vi "two_button.vi"(7 "callee":refnum<vi>, 8 "error in (no error)":errorcluster, 11 "configuration":T1) -> (0 "error out":errorcluster, 3 "dialog_selection":T2)   [LabVIEW 2015, in "lv-dialog-interfaces.lvlib"]
uses:
  lv-dialog-interfaces.lvlib
  <userlib>/antonio-alexander/lv-dialog/api/v1/public/_controls/selection.ctl
  private/_controls/dialog_type.ctl
  private/_controls/hmi_references.ctl
  private/_controls/configuration.ctl
  <vilib>/event_ctls.llb/eventvkey.ctl
  <userlib>/antonio-alexander/lv-dialog/api/v1/v1.lvlib
panel:
  out "dialog":string
  in  "button_1":bool
  in  "button_2":bool
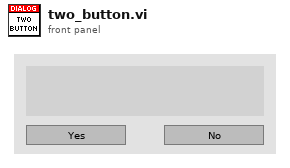
[diagram p1: front panel]
types:
  T1 = cluster{"dialog_text":string, "boolean_text_1":string, "boolean_text_2":string}
  T2 = typedef "lv-dialog.lvlib/v1.lvlib/selection.ctl" = enum16{"null", "panel_closed", "button_1", "button_2", "button_3", "cancelled"}
  T3 = typedef "lv-dialog-interfaces.lvlib/dialog_type.ctl" = enum16{"null", "one_button", "two_button", "three_button", "confirmation", "busy_wait", "error", "busy_wait_embed", "combo_box", "data_entry_string", "data_entry_numeric"}
  T4 = typedef "lv-dialog-interfaces.lvlib/configuration.ctl" = cluster{"dialog_text":string, "boolean_text_1":string, "boolean_text_2":string, "boolean_text_3":string, "inner_color":u32, "outer_color":u32, "wait_s":dbl, "error_status":bool, "error_source":string, "error_details":string, "string []":string[], "custom_entry":bool}
  T5 = typedef "lv-dialog-interfaces.lvlib/hmi_references.ctl" = cluster{"vi_reference":refnum<vi>, "caller":refnum<vi>, "dialog":refnum<vi>, "button_1":refnum<vi>, "button_2":refnum<vi>, "button_3":refnum<vi>, "busy":refnum<vi>, "error_glyph":refnum<vi>, "error_source":refnum<vi>, "error_text":refnum<vi>, "combo_box":refnum<vi>}
  T6 = typedef "eventvkey.ctl" = enum16{"ASCII", "Enter", "Return", "Shift", "Ctrl", "Alt", "Cmd", "Opt", "Caps", "NumLock", "Clear", "Break", "Up", "Down", "Left", "Right", "Insert", "Delete", "Home", "End", "PageUp", "PageDown", "Escape", "Help", "Pause", "ScrollLock", "F1", "F2", "F3", "F4", "F5", "F6", "F7", "F8", "F9", "F10", "F11", "F12", "F13", "F14", "F15", "F16", "F17", "F18", "F19", "F20", "F21", "F22", "F23", "F24", "Play", "VolumeUp", "VolumeDown", "Mute", "Two Byte Char"}
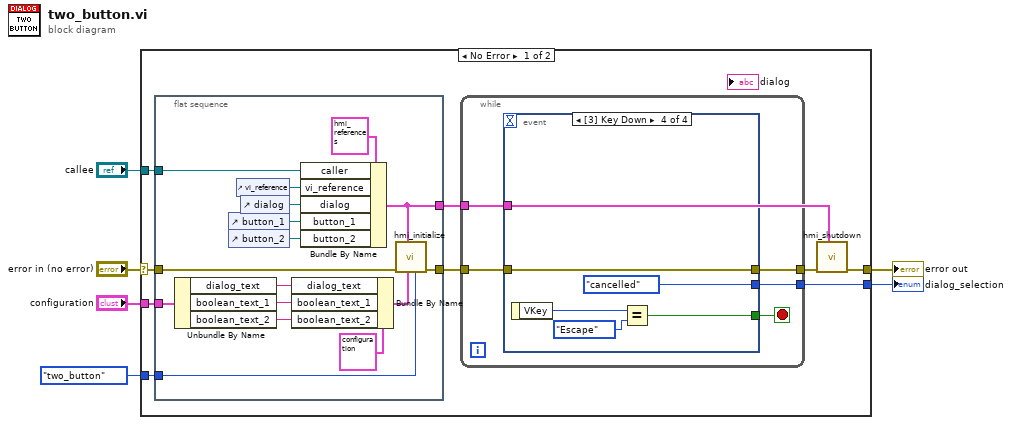
[diagram p0: block diagram]
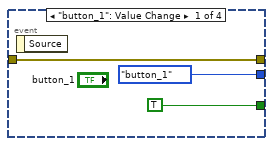
[diagram p2: hidden frame]
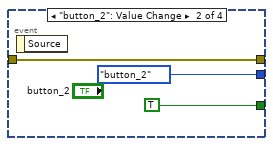
[diagram p3: hidden frame]
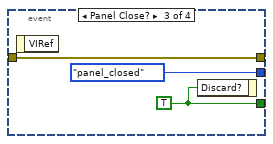
[diagram p4: hidden frame]
diagram:
  n1 = case shown="No Error" "error in (no error)" {
    selector: "error in (no error)" -> [w15 w51]
    tunnel: dialog_type."two_button" ("dialog_type") -> [w14 _]
    tunnel: [w12 _] -> w4
    tunnel: "callee" -> [w11 _]
    tunnel: [w9 w51] -> w2
    tunnel: "configuration" -> [w8 _]
    frame No Error {
      n2 = flat-sequence {
        tunnel: w15 -> [w24]
        tunnel: w14 -> [w27]
        tunnel: [w26] -> w13
        tunnel: w11 -> [w23]
        tunnel: [w22] -> w7
        tunnel: w8 -> [w20]
        frame #0 {
          n3 = Unbundle By Name(w20) -> ("dialog_text"=w18:string, "boolean_text_1"=w17:string, "boolean_text_2"=w16:string)
          n4 = control-ref of="button_1"() -> (w29:refnum<vi>)
          n5 = control-ref of="button_2"() -> (w25:refnum<vi>)
          n6 = control-ref of="vi_reference"() -> (w31:refnum<vi>)
          n7 = control-ref of="dialog"() -> (w30:refnum<vi>)
          n8 = Bundle By Name(cluster=T4 {"dialog_text"="", "boolean_text_1"="", "boolean_text_2"="", "boolean_text_3"="", "inner_color"=16711680, "outer_color"=6618880, "wait_s"=nan, "error_status"=FALSE, "error_source"="", "error_details"="", "string []"=[], "custom_entry"=FALSE} ("configuration"), "dialog_text"=w18, "boolean_text_1"=w17, "boolean_text_2"=w16) -> (w19:T4)
          n9 = Bundle By Name(cluster=T5 {"vi_reference"=refnum, "caller"=refnum, "dialog"=refnum, "button_1"=refnum, "button_2"=refnum, "button_3"=refnum, "busy"=refnum, "error_glyph"=refnum, "error_source"=refnum, "error_text"=refnum, "combo_box"=refnum}, "caller"=w23, "vi_reference"=w31, "dialog"=w30, "button_1"=w29, "button_2"=w25) -> (w22:T5)
          n10 = call "hmi_initialize.vi"("dialog_type"=w27, "configuration"=w19, "references"=w22, "error in (no error)"=w24) -> ("error out"=w26:errorcluster)  [unwired: 7 in]
        }
      }
      n11 = while {
        tunnel: [w34] -> w12
        tunnel: w13 -> [w36]
        tunnel: [w35] -> w10
        tunnel: w7 -> [w32]
        stop <- w33 stop-if-true
        n12 = event shown="[3] Key Down" {
          selector: _ -> [_ _ _ _]
          dyn-events: _ -> [_ _ _ _]
          timeout: _ -> [_ _ _ _]
          tunnel: w36 -> [w39 w42 w45 w50]
          tunnel: [w39 w42 w45 w50] -> w35
          tunnel: [selection."button_1" ("dialog_selection") selection."button_2" ("dialog_selection") selection."panel_closed" ("dialog_selection") selection."cancelled" ("dialog_selection")] -> w34
          tunnel: w32 -> [_ _ _ _]
          tunnel: [TRUE ("Discard?") TRUE ("Discard?") w43 w48] -> w33
          event "button_1": Value Change {
            n13 = event-data() -> ()  [unwired: 1 in, 1 out]
          }
          event "button_2": Value Change {
            n14 = event-data() -> ()  [unwired: 1 in, 1 out]
          }
          event Panel Close? {
            w43 = TRUE ("Discard?")
            n15 = event-data() -> ()  [unwired: 1 in, 1 out]
            n16 = event-data("Discard?"=w43) -> ()  [unwired: 1 in, 1 out]
          }
          event Key Down {
            n17 = event-data() -> ("VKey"=w47:T6)  [unwired: 1 in]
            n18 = Equal?(x=w47, y=eventvkey."Escape" ("VKey")) -> (x = y?=w48:bool)
          }
        }
      }
      n19 = call "hmi_shutdown.vi"("references"=w7, "error in (no error)"=w10) -> ("error out"=w9:errorcluster)  [unwired: 9 in]
    }
    frame Error {
    }
  }
  "error out" <- w2
  "dialog_selection" <- w4
